vi "closeResource.vi"(8 "error in (no error)":errorcluster, 11 "SR430Class in":refnum<class "SR430Class.lvclass">) -> (0 "error out":errorcluster, 3 "SR430Class out":refnum<class "SR430Class.lvclass">)   [LabVIEW 2015, in "SR430Class.lvclass"]
uses:
  class/SR430Class.lvclass
  class/SR430Class.lvclass/SR430Class.ctl
  support/SR430 Driver/SR430Driver.lvlib
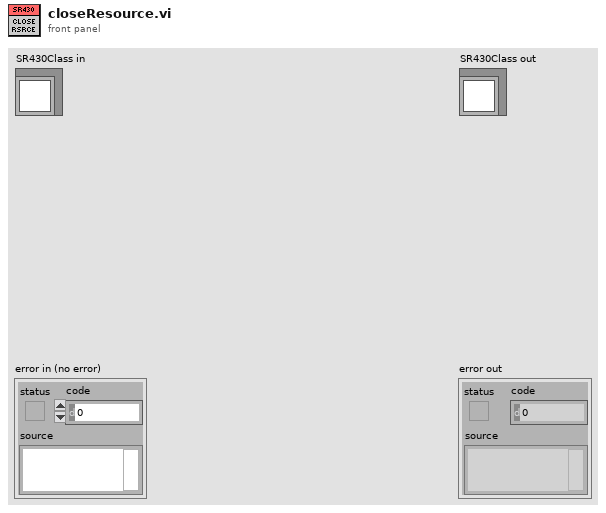
[diagram p1: front panel]
types:
  T1 = typedef "SR430Driver.lvlib/SR430_VISA Control.ctl" = cluster{"VISA resource name":refnum<visa-resource-name>}
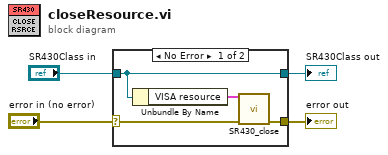
[diagram p0: block diagram]
diagram:
  n1 = case shown="No Error" "error in (no error)" {
    selector: "error in (no error)" -> [w6 w10]
    tunnel: [w5 w10] -> w3
    tunnel: [w8 w9] -> w1
    tunnel: "SR430Class in" -> [w8 w9]
    frame No Error {
      n2 = Unbundle By Name(w8) -> ("VISA resource"=w7:T1)
      n3 = call "SR430_close.vi"("SR430 VISA Cluster"=w7, "error in (no error)"=w6) -> ("error out"=w5:errorcluster)  [unwired: 13 in]
    }
    frame Error {
    }
  }
  "error out" <- w3
  "SR430Class out" <- w1
